vi "Util_Array_PoseWCurv_to_XY.vi"(11 "inArrayPoseWCurve":T1[](array[typedef])) -> (3 "outArrayXY":cluster{dbl[], dbl[]})   [LabVIEW 2019, in "Trajectory_Library.lvlib"]
doc: "This is a convience function to convert the X, Y portions of a PoseWithCurvature array into arrays of X,Y for charting."
uses:
  Trajectory_Library.lvlib
  POSEwCURVATURE.ctl
  POSE2D.ctl
  TRANSLATION2D.ctl
  ROTATION2D.ctl
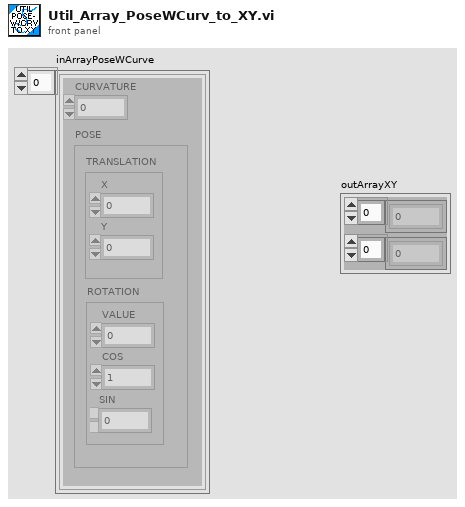
[diagram p1: front panel]
types:
  T1 = typedef "Trajectory_Library.lvlib/POSEwCURVATURE.ctl" = cluster{"CURVATURE":dbl, "POSE":T2}
  T2 = typedef "Trajectory_Library.lvlib/POSE2D.ctl" = cluster{"TRANSLATION":T3, "ROTATION":T4}
  T3 = typedef "Trajectory_Library.lvlib/TRANSLATION2D.ctl" = cluster{"X":dbl, "Y":dbl}
  T4 = typedef "Trajectory_Library.lvlib/ROTATION2D.ctl" = cluster{"VALUE":dbl, "COS":dbl, "SIN":dbl}
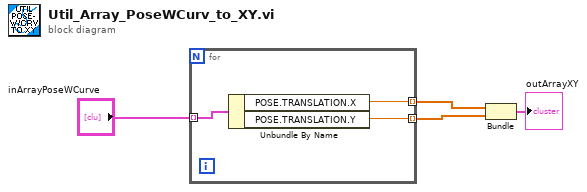
[diagram p0: block diagram]
diagram:
  n1 = for {
    tunnel: [w7] -> w3 mode=indexing
    tunnel: [w6] -> w4 mode=indexing
    tunnel: "inArrayPoseWCurve" -> [w5] mode=indexing
    n2 = Unbundle By Name(w5) -> ("POSE.TRANSLATION.X"=w7:dbl, "POSE.TRANSLATION.Y"=w6:dbl)
  }
  n3 = Bundle(w3, w4) -> (→"outArrayXY":cluster{dbl[], dbl[]})  [unwired: 1 in]
